vi "GetNet-Client Send Message.vi"(8 "error in":errorcluster, 9 "Send via Network Argument":T1, 11 "Data Cluster in":T2) -> (0 "error out":errorcluster, 3 "Data Cluster out":T2)   [LabVIEW 2014, in "GenNet-Client.lvlib"]
doc: "Checks the TCP network connection, writes the message out, waits for the reply from the server and reports the response and/or an error to the parent (caller)."
uses:
  GenNet-Client.lvlib
  Module Data--cluster.ctl
  Send via Network Argument--cluster.ctl
  <vilib>/Utility/error.llb/Clear Errors.vi
  GenNet Version-Safe Unflatten Variant.vi
  hse-gennet.lvlib
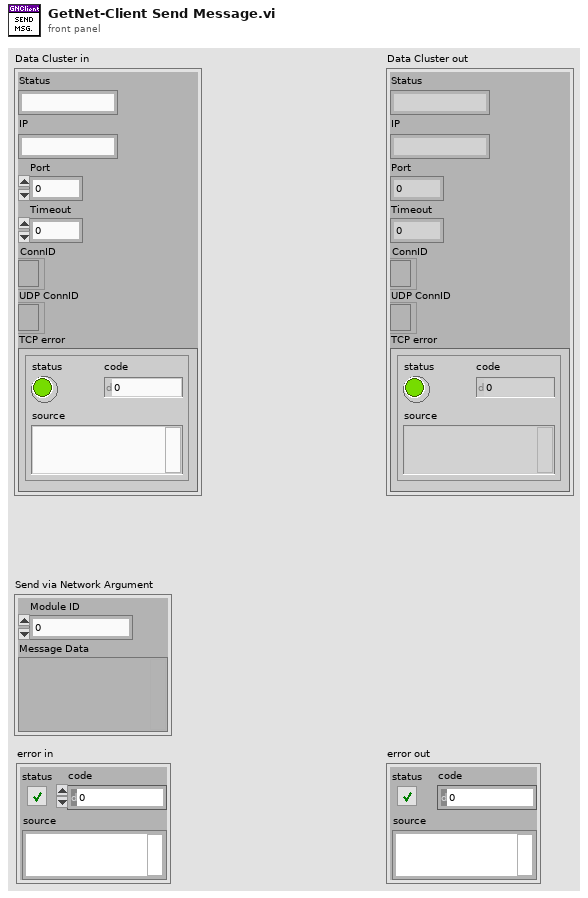
[diagram p1: front panel]
types:
  T1 = typedef "GenNet-Client.lvlib/Send via Network Argument--cluster.ctl" = cluster{"Module ID":i32, "Message Data":variant}
  T2 = typedef "GenNet-Client.lvlib/Module Data--cluster.ctl" = cluster{"Status":string, "IP":string, "Port":u16, "Timeout":i32, "ConnID":refnum<k5>, "UDP ConnID":refnum<k16>, "TCP error":errorcluster}
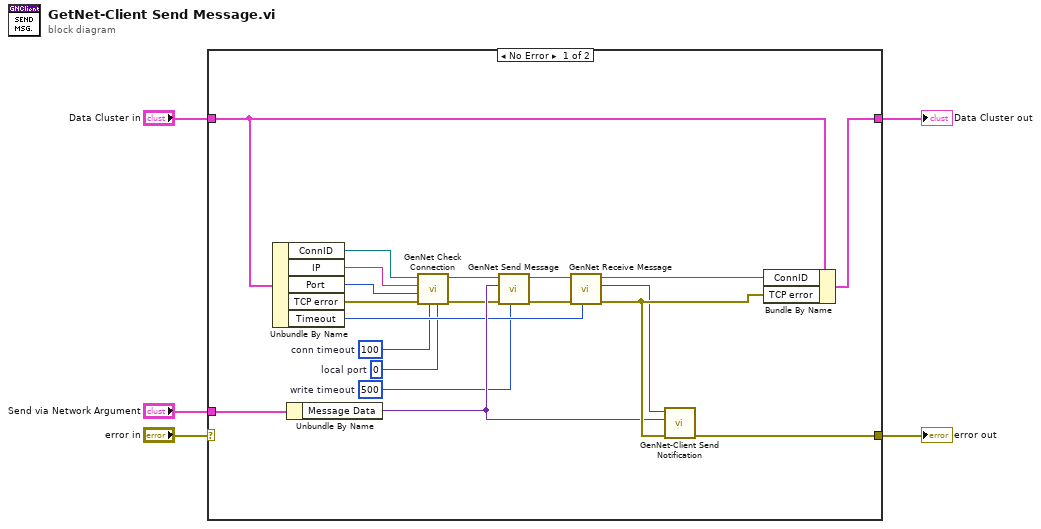
[diagram p0: block diagram]
diagram:
  n1 = case shown="No Error" "error in" {
    selector: "error in" -> [_ w27]
    tunnel: [w6 w27] -> w5
    tunnel: [w9 w26] -> w4
    tunnel: "Data Cluster in" -> [w8 w26]
    tunnel: "Send via Network Argument" -> [w7 _]
    frame No Error {
      w20 = 500  # write timeout
      w19 = u16 0  # local port
      w18 = 100  # conn timeout
      n2 = Unbundle By Name(w8) -> ("ConnID"=w13:refnum<k5>, "IP"=w16:string, "Port"=w17:u16, "TCP error"=w25:errorcluster, "Timeout"=w21:i32)
      n3 = Unbundle By Name(w7) -> ("Message Data"=w22:variant)
      n4 = call "GenNet Check Connection.vi"("local port (0)"=w19, "timeout [ms]"=w18, "error in (no error)"=w25, "remote port"=w17, "ip address"=w16, "TCP Network Connection in"=w13) -> ("error out"=w15:errorcluster, "TCP Network Connection out"=w14:refnum<k5>)  [unwired: 4 in]
      n5 = call "GenNet Send Message.vi"("timeout [ms]"=w20, "error in (no error)"=w15, "Message Data"=w22, "TCP Network Connection in"=w14) -> ("error out"=w12:errorcluster, "TCP Network Connection out"=w10:refnum<k5>)  [unwired: 6 in]
      n6 = call "GenNet Receive Message.vi"("timeout [ms]"=w21, "error in (no error)"=w12, "TCP Network Connection in"=w10) -> ("error out"=w24:errorcluster, "Message Data"=w23:variant, "TCP Network Connection out"=w11:refnum<k5>)  [unwired: 6 in]
      n7 = call "GenNet-Client Send Notification.vi"("error in"=w24, "Original Message Data"=w22, "Received Message Data"=w23) -> ("error out"=w6:errorcluster)  [unwired: 8 in]
      n8 = Bundle By Name(cluster=w8, "ConnID"=w11, "TCP error"=w24) -> (w9:T2)
    }
    frame Error {
    }
  }
  "error out" <- w5
  "Data Cluster out" <- w4
